vi "GetCommands.vi"(9 "Script Number":i32) -> (0 "Script Exists":bool, 2 "Commands":string[](array[string]), 3 "Camera Settings":dbl[](array[numeric]), 5 "Data Interval (s)":dbl)   [LabVIEW 2018]
panel:
  out "error out":errorcluster
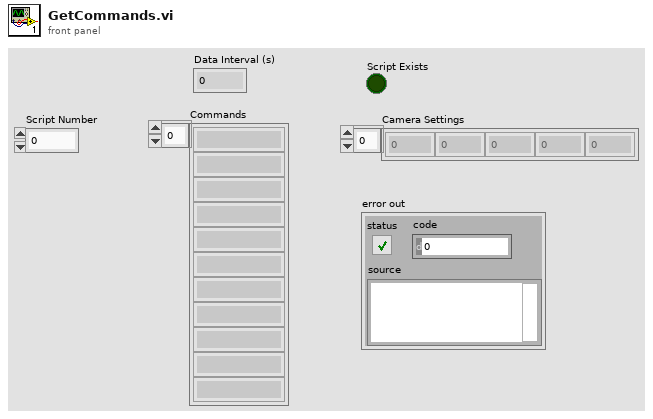
[diagram p1: front panel]
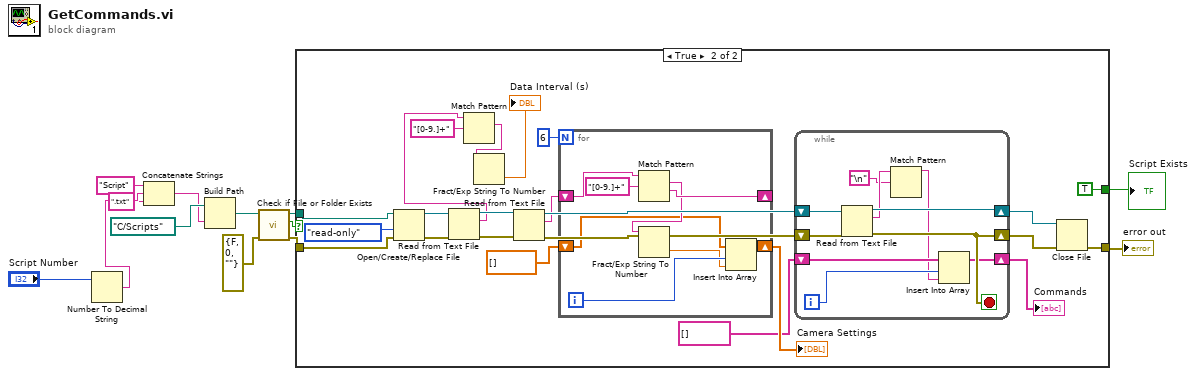
[diagram p0: block diagram]
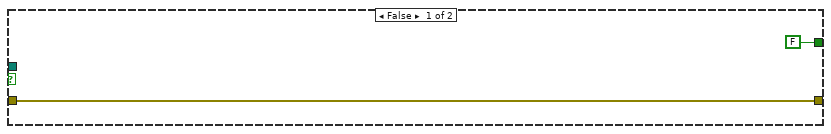
[diagram p2: hidden frame]
diagram:
  n1 = Number To Decimal String(number="Script Number") -> (decimal integer string=w10:string)  [unwired: 1 in]
  n2 = Concatenate Strings("Script" ("string"), w10, ".txt" ("string")) -> (w11:string)
  n3 = Build Path(base path=path "C:/Scripts" ("file path (use dialog)"), name or relative path=w11) -> (appended path=w9:path)
  n4 = call <vilib>:"Check if File or Folder Exists.vi"("error in (no error)"=errorcluster {"status"=FALSE, "code"=0, "source"=""} ("error in"), "path"=w9) -> ("error out"=w5:errorcluster, "file or folder exists?"=w7:bool, "dup path"=w6:path)  [unwired: 7 in]
  n5 = case shown="True" w7 {
    tunnel: w6 -> [_ w37]
    tunnel: w5 -> [w15 w36]
    tunnel: [w15 w35] -> w3
    tunnel: [FALSE ("Boolean") TRUE ("Boolean")] -> w1
    frame False {
    }
    frame True {
      n6 = Open/Create/Replace File(file path (use dialog)=w37, error in=w36, access (0:read/write)=enum16{"read/write", "read-only", "write-only"}."read-only") -> (refnum out=w21:refnum<file>, error out=w23:errorcluster)  [unwired: 3 in, 1 out]
      n7 = Read from Text File(file (use dialog)=w21, error in=w23) -> (refnum out=w20:refnum<file>, text=w18:string, error out=w22:errorcluster)  [unwired: 2 in, 1 out]
      n8 = Match Pattern(string=w18, regular expression="[0-9.]+") -> (match substring=w17:string)  [unwired: 1 in, 3 out]
      n9 = Fract/Exp String To Number(string=w17) -> (number=→"Data Interval (s)":dbl)  [unwired: 3 in, 1 out]
      n10 = Read from Text File(file (use dialog)=w20, error in=w22) -> (refnum out=w33:refnum<file>, text=w30:string, error out=w34:errorcluster)  [unwired: 2 in, 1 out]
      n11 = for {
        N: 6 -> [_]
        shift-right: [w44] -> _
        shift-left: w30 -> [w46]
        shift-right: [w40] -> w28
        shift-left: dbl[] [] -> [w39]
        i -> [w42]
        n12 = Match Pattern(string=w46, regular expression="[0-9.]+") -> (match substring=w43:string, after substring=w44:string)  [unwired: 1 in, 2 out]
        n13 = Fract/Exp String To Number(string=w43) -> (number=w41:dbl)  [unwired: 3 in, 1 out]
        n14 = Insert Into Array(array=w39, index=w42, new element=w41) -> (w40:dbl[])
      }
      "Camera Settings" <- w28
      n15 = while {
        shift-right: [w54] -> w32
        shift-left: w33 -> [w55]
        shift-right: [w53] -> w31
        shift-left: w34 -> [w56]
        shift-right: [w51] -> w27
        shift-left: string[] [] -> [w50]
        i -> [w52]
        stop <- w53 stop-if-true
        n16 = Read from Text File(file (use dialog)=w55, error in=w56) -> (refnum out=w54:refnum<file>, text=w49:string, error out=w53:errorcluster)  [unwired: 2 in, 1 out]
        n17 = Match Pattern(string=w49, regular expression="\n") -> (before substring=w48:string)  [unwired: 1 in, 3 out]
        n18 = Insert Into Array(array=w50, index=w52, new element=w48) -> (w51:string[])
      }
      "Commands" <- w27
      n19 = Close File(refnum=w32, error in=w31) -> (error out=w35:errorcluster)  [unwired: 1 out]
    }
  }
  "error out" <- w3
  "Script Exists" <- w1
